vi "NI XNET CAN Signal Logger - Configure Dialog.vi"(8 "error in (no error)":errorcluster, 10 "CAN Configurations in":T1[](array[typedef]) {"Sample Rate (Hz)" format="%#_13g"}, 11 "LogSpec in":T2={"Log file folder"=path "C:/Users/NI/Desktop/Data", "Log file name"="LogFile_{Year}-{Month}-{Day}-{Hour}-{Minute}-{Second}.tdms", "Segment Files"=FALSE, "Segment File Size"=100} {"Segment File Size" format="%.0f MB"}) -> (0 "error out":errorcluster, 2 "CAN Configurations out":T1[](array[typedef]) {"Sample Rate (Hz)" format="%#_13g"}, 3 "LogSpec out":T2={"Log file folder"=path "C:/Users/NI/Desktop/Data", "Log file name"="LogFile_{Year}-{Month}-{Day}-{Hour}-{Minute}-{Second}.tdms", "Segment Files"=FALSE, "Segment File Size"=100} {"Segment File Size" format="%.0f MB"})   [LabVIEW 2021, in "XNET-CAN-Signal-Logger.lvlib"]
uses:
  XNET-CAN-Signal-Logger.lvlib
  Typedef/Def-CAN Port Configuration.ctl
  Typedef/Def-LogSpec.ctl
  <resource>/objmgr/xnet.rc
panel:
  in  "OK":bool
  in  "CAN Configurations":T1[](array[typedef]) {"Sample Rate (Hz)" format="%#_13g"}
  out "Preview":string caption="Preview:"
  in  "Log file name":string="LogFile_{Year}-{Month}-{Day}-{Hour}-{Minute}-{Second}.tdms"
  in  "Log file folder":path=path "C:/Users/NI/Desktop/Data"
  in  "Cancel":bool
  in  "Segment Files":bool=TRUE
  in  "Segment File Size":i64=100 caption="Seg File Size" format="%.0f MB"
  # "Configuration"
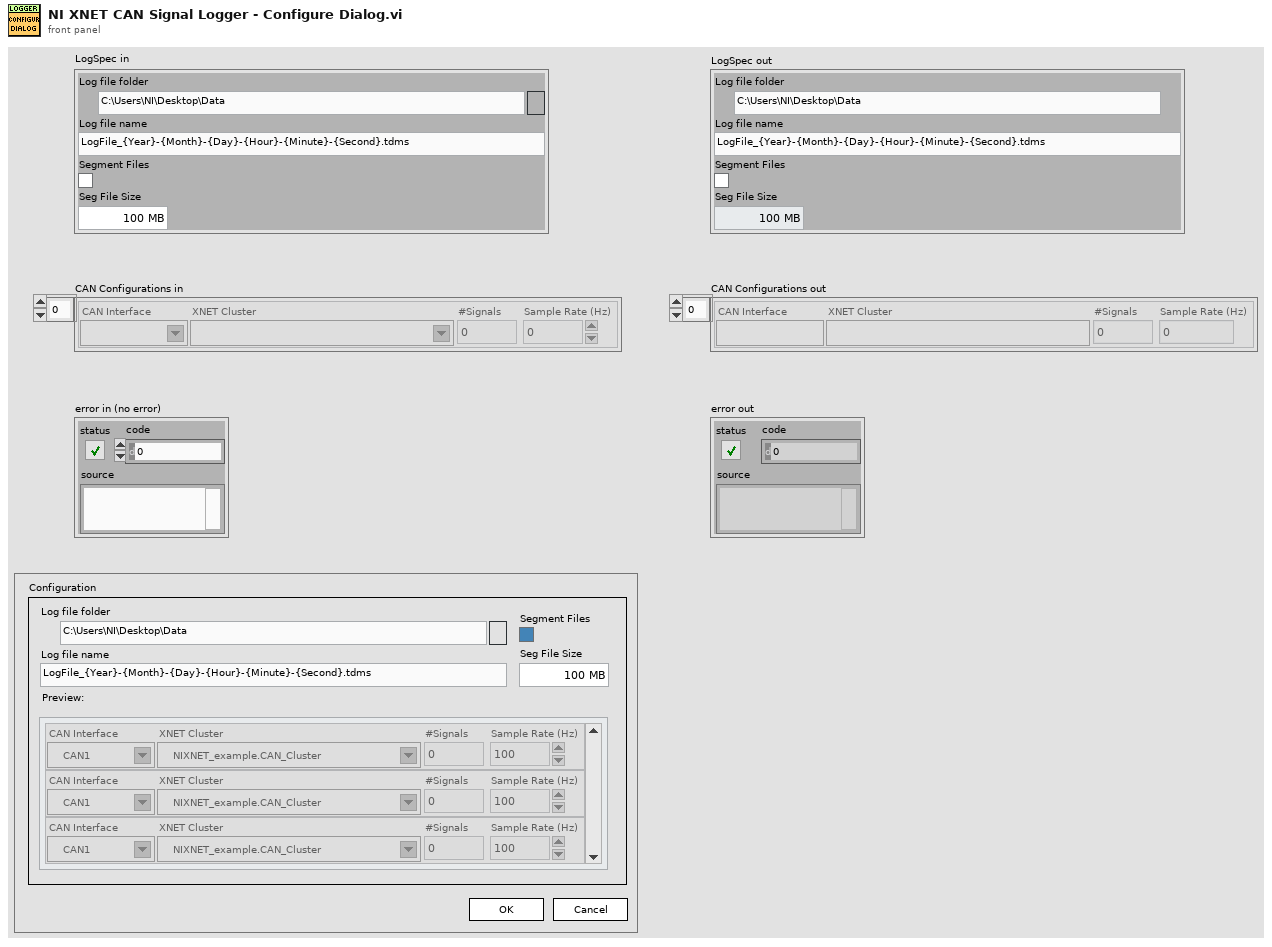
[diagram p1: front panel]
types:
  T1 = typedef "XNET-CAN-Signal-Logger.lvlib/Def-CAN Port Configuration.ctl" = cluster{"CAN Interface":refnum<k21>, "XNET Cluster":refnum<k21>, "#Signals":i32, "Sample Rate (Hz)":dbl}
  T2 = typedef "XNET-CAN-Signal-Logger.lvlib/Def-LogSpec.ctl" = cluster{"Log file folder":path, "Log file name":string, "Segment Files":bool, "Segment File Size":i64}
  T3 = enum32{"Invalid", "Standard", "Closed", "Hidden", "Minimized", "Maximized"}
  T4 = enum32{"invalid app kind", "Development System", "Run Time System", "Student Edition", "Embedded LabVIEW", "Evaluation", "Custom"}
  T5 = cluster{"Core":cluster{"Current VI Reference":refnum<vi>, "Close Panel on Exit?":bool}, "LogSpec in":T2, "CAN Configurations in":T1[]}
  T6 = cluster{"Current VI Reference":refnum<vi>, "Close Panel on Exit?":bool}
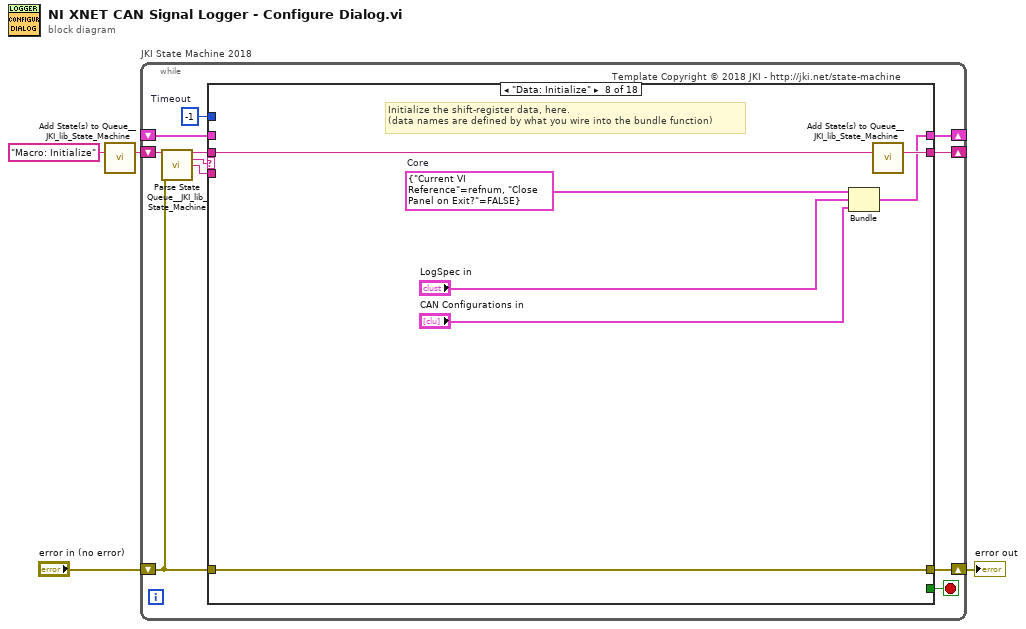
[diagram p0: block diagram]
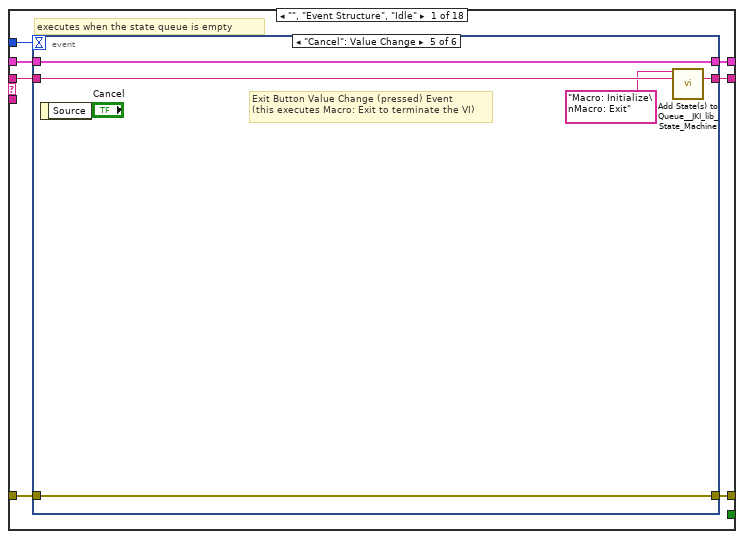
[diagram p2: hidden frame]
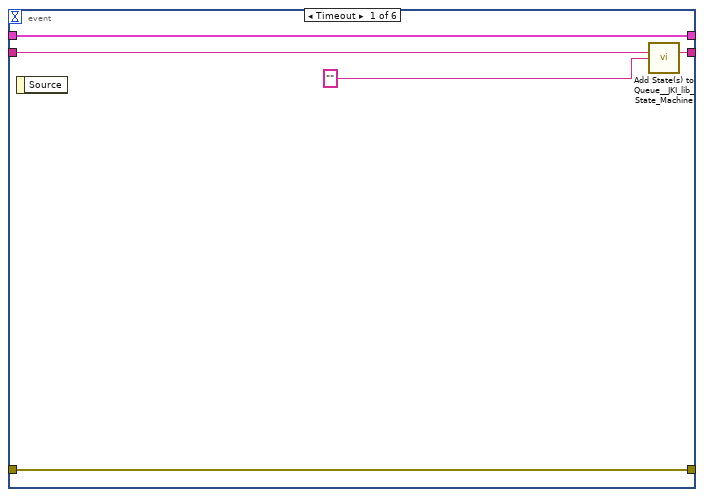
[diagram p3: hidden frame]
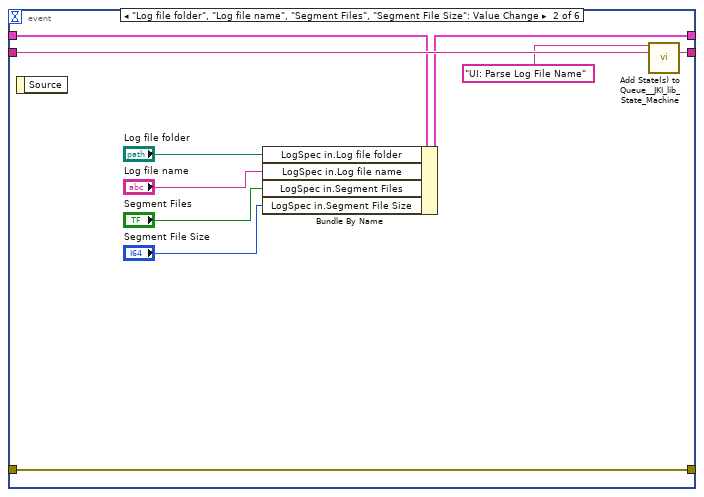
[diagram p4: hidden frame]
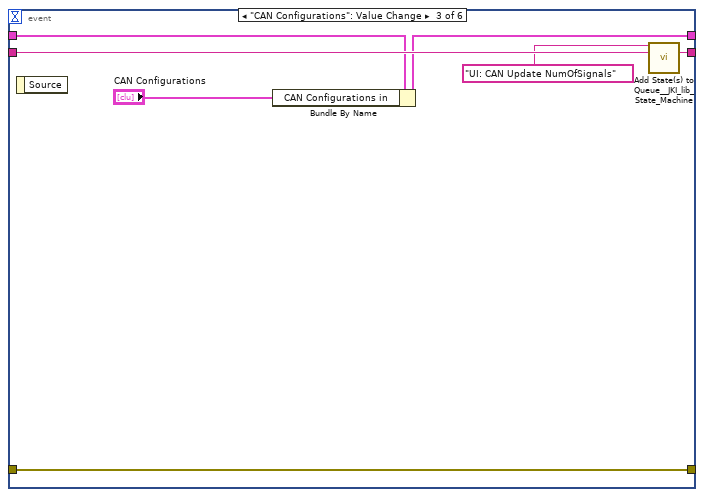
[diagram p5: hidden frame]
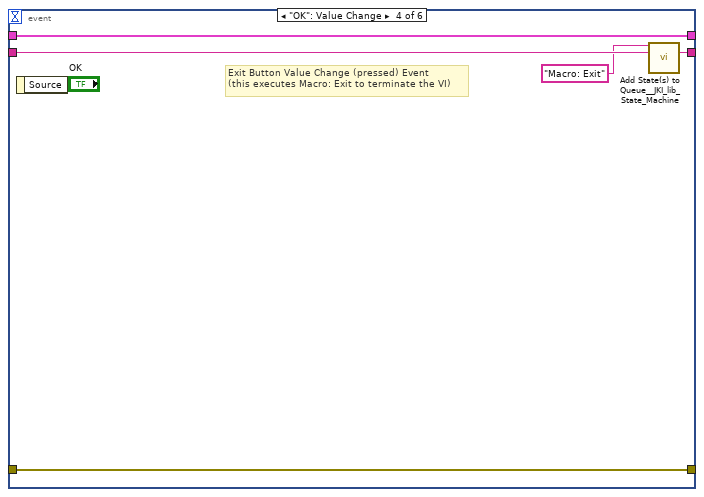
[diagram p6: hidden frame]
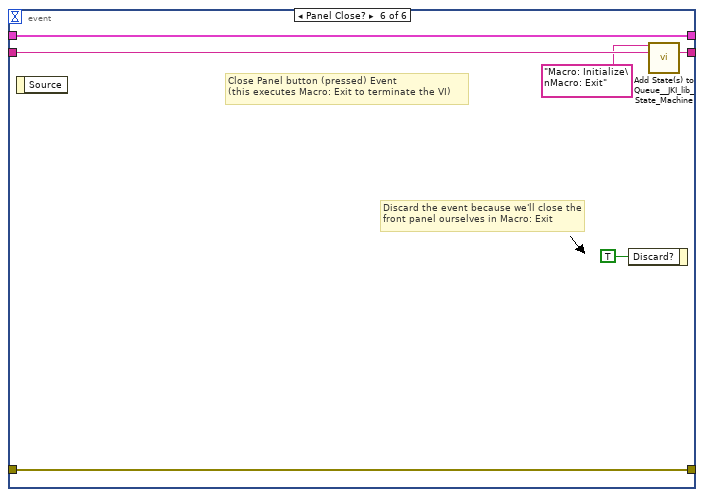
[diagram p7: hidden frame]
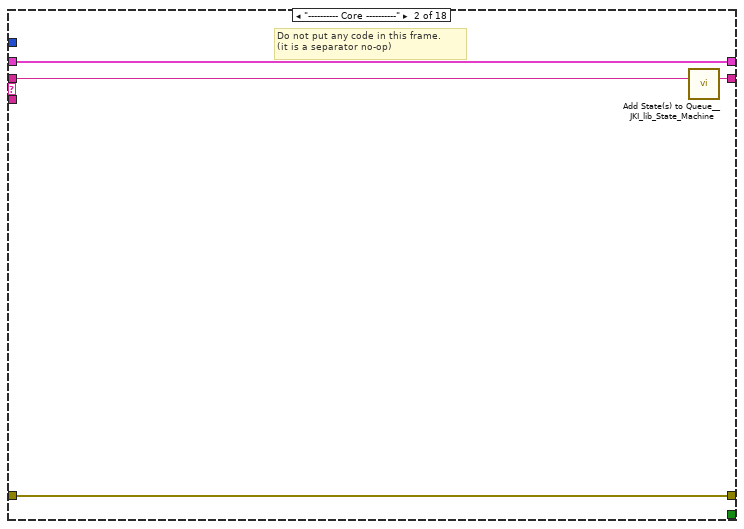
[diagram p8: hidden frame]
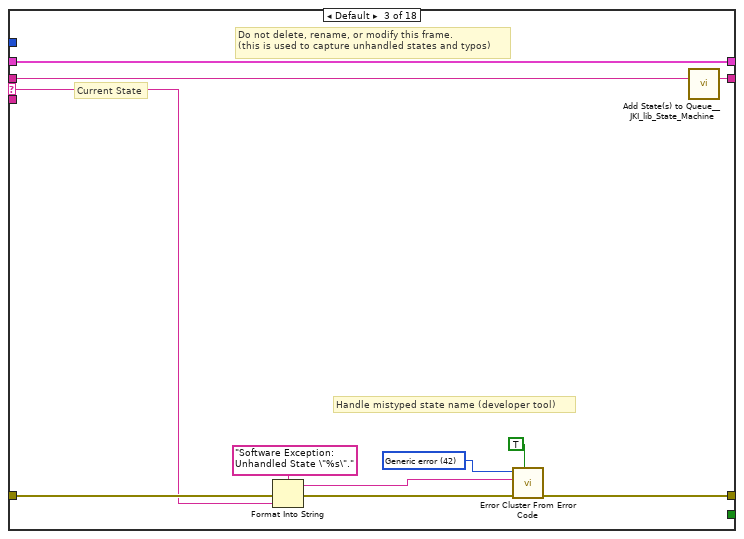
[diagram p9: hidden frame]
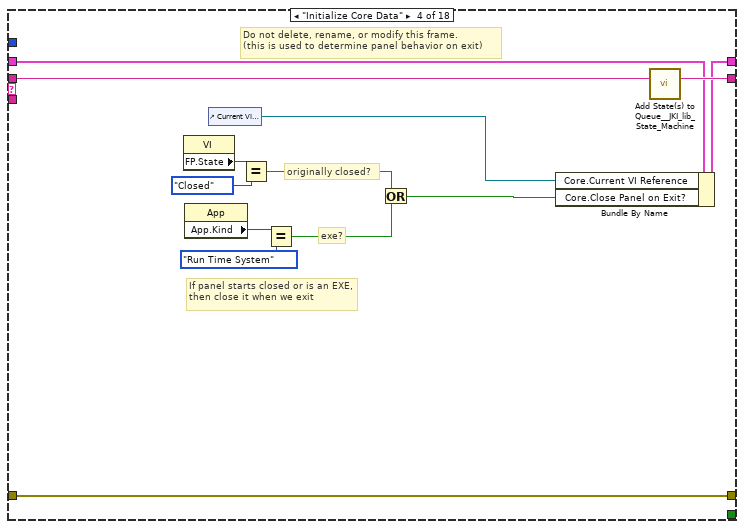
[diagram p10: hidden frame]
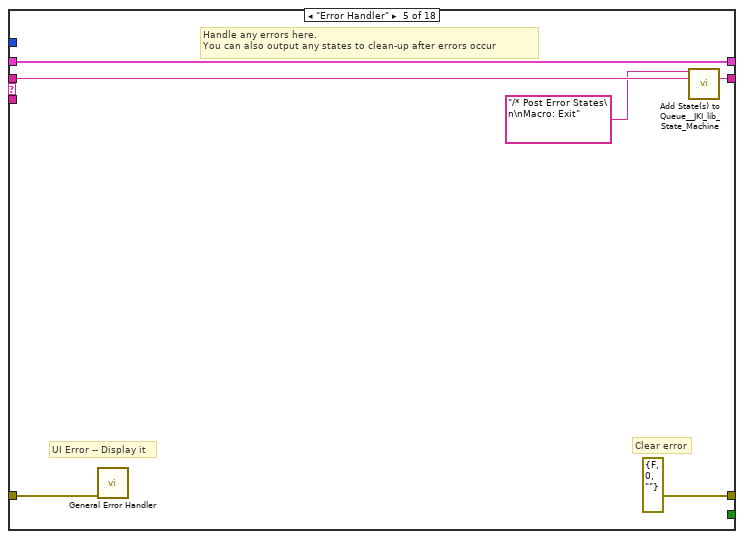
[diagram p11: hidden frame]
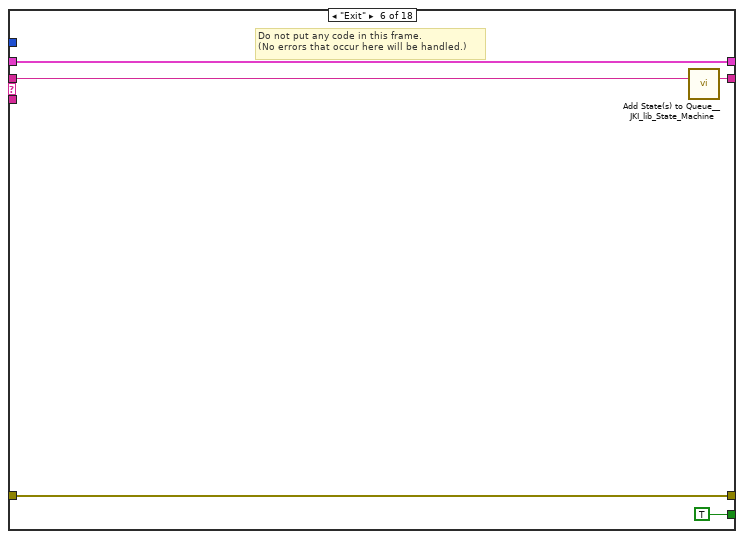
[diagram p12: hidden frame]
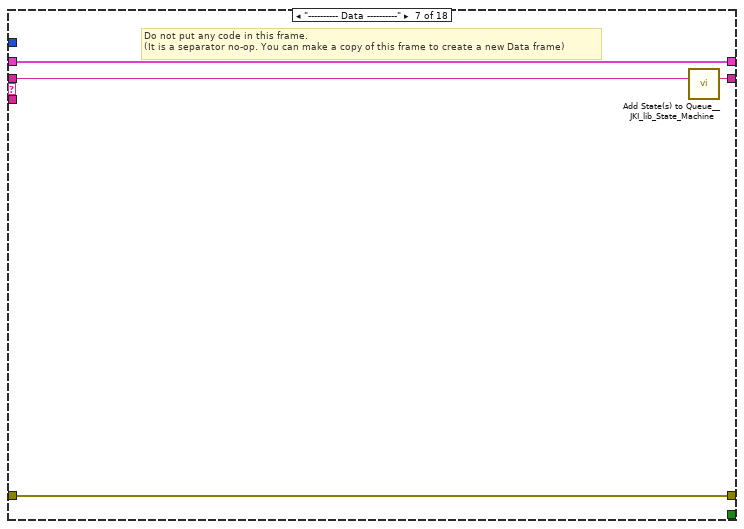
[diagram p13: hidden frame]
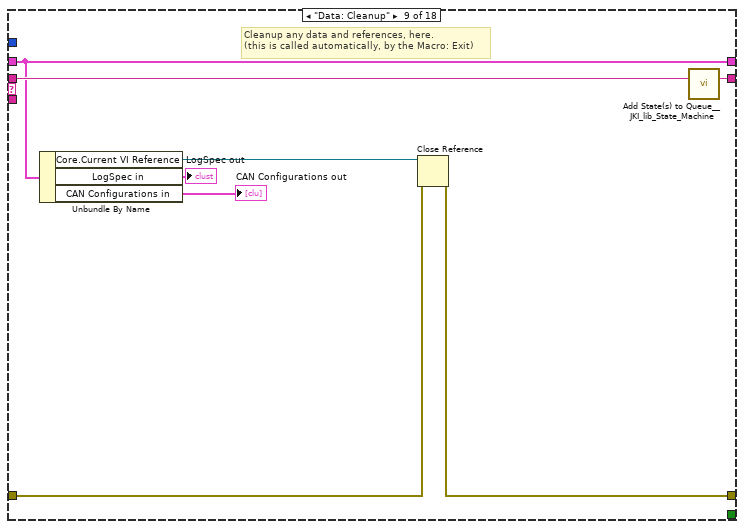
[diagram p14: hidden frame]
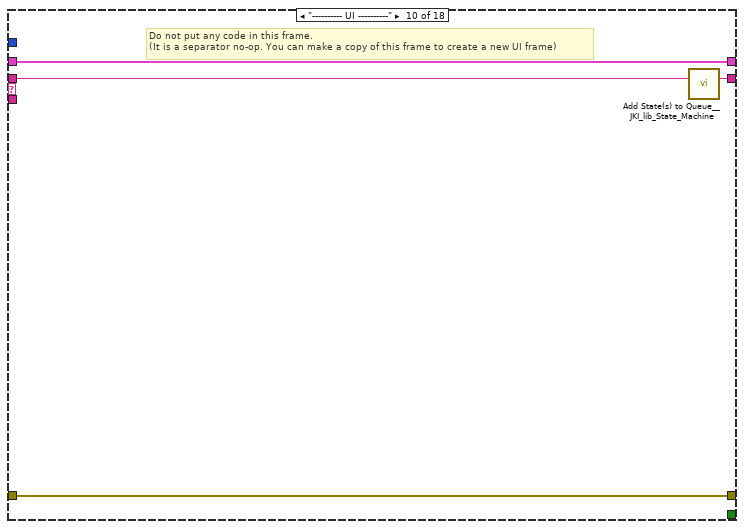
[diagram p15: hidden frame]
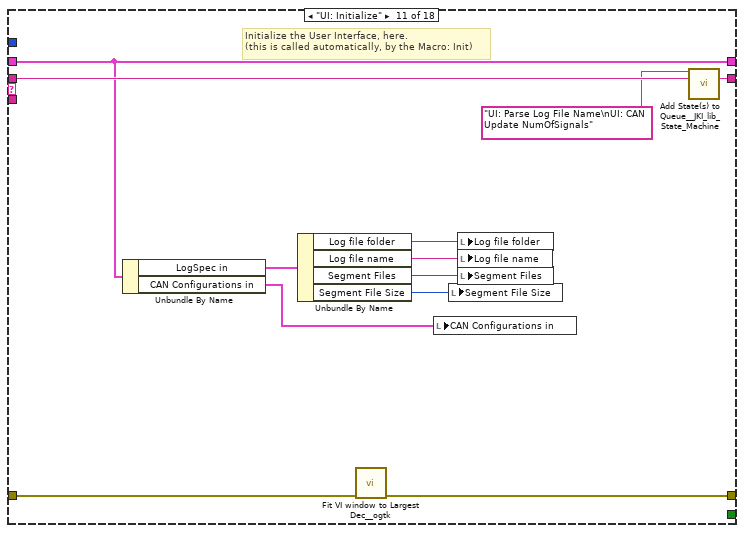
[diagram p16: hidden frame]
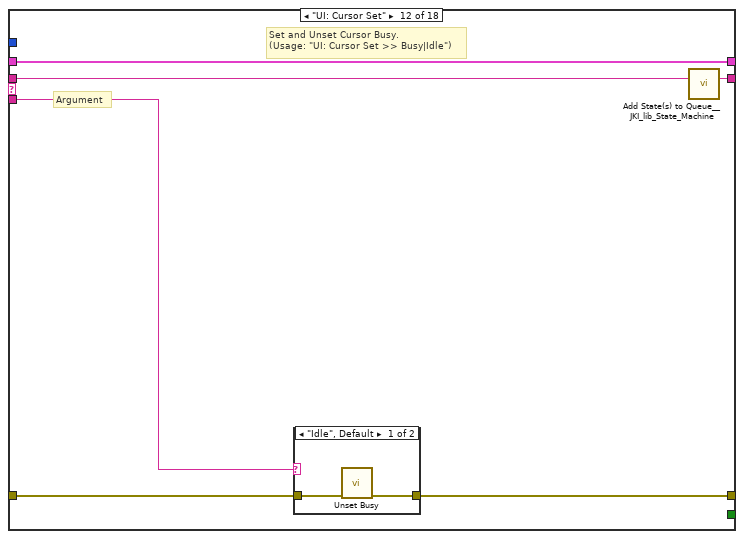
[diagram p17: hidden frame]
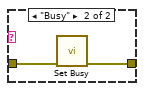
[diagram p18: hidden frame]
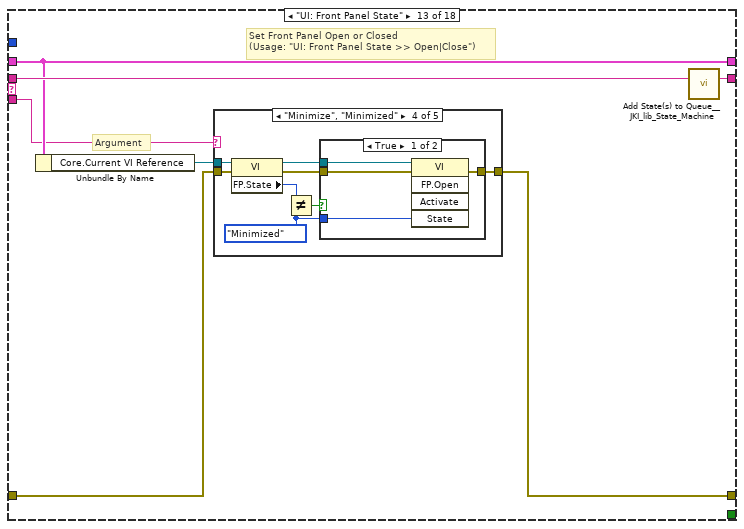
[diagram p19: hidden frame]
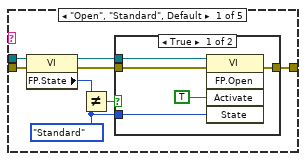
[diagram p20: hidden frame]
diagram:
  n1 = call <vilib>:"Add State(s) to Queue__JKI_lib_State_Machine.vi"("State(s) in (\"\")"="Macro: Initialize") -> ("States Out"=w4:string)  [unwired: 14 in]
  n2 = while "JKI State Machine 2018" {
    shift-right: [w8] -> _
    shift-left: _ -> [w7]
    shift-right: [w11] -> w1
    shift-left: "error in (no error)" -> [w5]
    shift-right: [w10] -> _
    shift-left: w4 -> [w12]
    stop <- w9 stop-if-true
    w6 = -1  # Timeout
    # "Template Copyright © 2018 JKI - http://jki.net/state-machine"
    n3 = call <vilib>:"Parse State Queue__JKI_lib_State_Machine.vi"("State Queue"=w12, "Error In (no error)"=w5) -> ("Remaining States"=w14:string, "Current State"=w15:string, "Arguments"=w13:string)  [unwired: 11 in]
    n4 = case shown="\"Data: Initialize\"" w15 {
      selector: w15 -> [_ _ w65 _ _ _ _ _ _ _ _ _ _ _ _ _ _ _]
      tunnel: w14 -> [w22 w64 w69 w88 w94 w99 w103 w110 w118 w122 w134 w140 w151 w222 w229 w238 w243 w253]
      tunnel: w13 -> [_ _ _ _ _ _ _ _ _ _ _ w135 w145 _ _ _ _ _]
      tunnel: w7 -> [w20 w61 w67 w81 w91 w97 w100 _ w113 w119 w126 w138 w147 w218 w224 w235 w240 w250]
      tunnel: [w19 w62 w71 w85 errorcluster {"status"=FALSE, "code"=0, "source"=""} ("error out") w96 w101 w107 w114 w120 w123 w136 w148 w220 w227 w236 w241 w251] -> w11
      tunnel: w5 -> [w18 w62 w70 w85 w90 w96 w101 w107 w115 w120 w132 w137 w149 w220 w227 w236 w241 w251]
      tunnel: [w21 w63 w68 w87 w93 w98 w102 w109 w117 w121 w133 w139 w150 w221 w228 w237 w242 w252] -> w10
      tunnel: [_ _ _ _ _ TRUE _ _ _ _ _ _ _ _ _ _ _ _] -> w9
      tunnel: [w17 w61 w67 w86 w91 w97 w100 w108 w113 w119 w126 w138 w147 w218 w226 w235 w240 w250] -> w8
      tunnel: w6 -> [w16 _ _ _ _ _ _ _ _ _ _ _ _ _ _ _ _ _]
      frame "", "Event Structure", "Idle" {
        # "executes when the state queue is empty"
        n5 = event shown="[4] \"Cancel\": Value Change" {
          selector: _ -> [_ _ _ _ _ _]
          dyn-events: _ -> [_ _ _ _ _ _]
          timeout: w16 -> [_ _ _ _ _ _]
          tunnel: w22 -> [w24 w37 w44 w49 w54 w60]
          tunnel: [w27 w36 w43 w48 w53 w59] -> w21
          tunnel: w20 -> [w25 w34 w41 w46 w51 w57]
          tunnel: [w26 w35 w42 w47 w52 w58] -> w19
          tunnel: w18 -> [w26 w35 w42 w47 w52 w58]
          tunnel: [w25 w32 w39 w46 w51 w57] -> w17
          event Timeout {
            n6 = event-data() -> ()  [unwired: 1 in, 1 out]
            n7 = call <vilib>:"Add State(s) to Queue__JKI_lib_State_Machine.vi"("State(s) in (\"\")"=w24, "State(s) at Back (\"\")"="" ("string")) -> ("States Out"=w27:string)  [unwired: 13 in]
          }
          event "Log file folder", "Log file name", "Segment Files", "Segment File Size": Value Change {
            n8 = event-data() -> ()  [unwired: 1 in, 1 out]
            n9 = Bundle By Name(cluster=w34, "LogSpec in.Log file folder"="Log file folder", "LogSpec in.Log file name"="Log file name", "LogSpec in.Segment Files"="Segment Files", "LogSpec in.Segment File Size"="Segment File Size") -> (w32:T5)
            n10 = call <vilib>:"Add State(s) to Queue__JKI_lib_State_Machine.vi"("State(s) in Front (\"\")"="UI: Parse Log File Name", "State(s) in (\"\")"=w37) -> ("States Out"=w36:string)  [unwired: 13 in]
          }
          event "CAN Configurations": Value Change {
            n11 = event-data() -> ()  [unwired: 1 in, 1 out]
            n12 = Bundle By Name(cluster=w41, "CAN Configurations in"="CAN Configurations") -> (w39:T5)
            n13 = call <vilib>:"Add State(s) to Queue__JKI_lib_State_Machine.vi"("State(s) in Front (\"\")"="UI: CAN Update NumOfSignals", "State(s) in (\"\")"=w44) -> ("States Out"=w43:string)  [unwired: 13 in]
          }
          event "OK": Value Change {
            # "Exit Button Value Change (pressed) Event\n(this executes Macro: Exit to terminate the VI)"
            n14 = event-data() -> ()  [unwired: 1 in, 1 out]
            n15 = call <vilib>:"Add State(s) to Queue__JKI_lib_State_Machine.vi"("State(s) in Front (\"\")"="Macro: Exit", "State(s) in (\"\")"=w49) -> ("States Out"=w48:string)  [unwired: 13 in]
          }
          event "Cancel": Value Change {
            # "Exit Button Value Change (pressed) Event\n(this executes Macro: Exit to terminate the VI)"
            n16 = event-data() -> ()  [unwired: 1 in, 1 out]
            n17 = call <vilib>:"Add State(s) to Queue__JKI_lib_State_Machine.vi"("State(s) in Front (\"\")"="Macro: Initialize\nMacro: Exit", "State(s) in (\"\")"=w54) -> ("States Out"=w53:string)  [unwired: 13 in]
          }
          event Panel Close? {
            # "Discard the event because we'll close the front panel ourselves in Macro: Exit"
            # "Close Panel button (pressed) Event\n(this executes Macro: Exit to terminate the VI)"
            n18 = event-data() -> ()  [unwired: 1 in, 1 out]
            n19 = event-data("Discard?"=TRUE) -> ()  [unwired: 1 in, 1 out]
            n20 = call <vilib>:"Add State(s) to Queue__JKI_lib_State_Machine.vi"("State(s) in Front (\"\")"="Macro: Initialize\nMacro: Exit", "State(s) in (\"\")"=w60) -> ("States Out"=w59:string)  [unwired: 13 in]
          }
        }
      }
      frame "---------- Core ----------" {
        # "Do not put any code in this frame.\n(it is a separator no-op)"
        n21 = call <vilib>:"Add State(s) to Queue__JKI_lib_State_Machine.vi"("State(s) in (\"\")"=w64) -> ("States Out"=w63:string)  [unwired: 14 in]
      }
      frame Default {
        w74 = 42 items=["No error", "Argument error", "Memory is full", "Out of zone", "End of file", "File already open", "Generic file I/O error", "File not found", "File permission error", "Disk is full", "Duplicate path", "Too many files open", "System feature not enabled", "Resource file not found", "Cannot add resource", "Resource not found", "Image not found", "Image memory error", "Pen does not exist", "Config type invalid", "Config token not found", "Config parse error", "Config memory error", "Bad external code format", "Bad external code offset", "External code not present", "Null window", "Destroy window error", "Null menu", "Print aborted", "Bad print record", "Print driver error", "Windows error during printing", "Memory error during printing", "Print dialog error", "Generic print error", "Invalid device refnum", "Device not found", "Device parameter error", "Device unit error", "Cannot open device", "Device call aborted", "Generic error", "Cancelled by user", "Object ID too low", "Object ID too high", "Object not in heap", "Unknown heap", "Unknown object (invalid DefProc)", "Unknown object (DefProc not in table)", "Message out of range", "Invalid (null) method", "Unknown message", "Manager call not supported", "Bad address", "Network operation in progress", "Network operation timed out", "Connection is busy", "Network attribute not supported", "Network error", "Address in use", "System out of memory", "Connection aborted", "Connection refused", "Not connected", "Already connected", "Connection closed", "Initialization error (interapplication manager)", "Bad occurrence", "Wait on unbound occurrence handler", "Occurrence queue overflow", "Datalog type conflict", "Unused", "Unrecognized type (interapplication manager)", "Memory corrupt", "Failed to make temporary DLL", "Old CIN version", "Drag socket not found", "Failed to load drop-object", "Failed to register OLE object", "Failed to release OLE object", "Format specifier type mismatch", "Unknown format specifier", "Too few format specifiers", "Too many format specifiers", "Scan failed", "Newer CIN version", "Error converting to variant", "Runtime menu error", "Password tampered", "Variant attribute not found", "Incompatible variant data type", "Event data is not available", "Event Store is not present", "Occurrence is not found", "Event Queue is not created", "Event info is not available", "Refnum passed is NULL", "Error retrieving Class GUID", "Error retrieving CoClass GUID", "Error retrieving TypeLib GUID.", "Bad built application magic bytes.", "Specific driver is different from the specific driver associated with the Logical Name.", "There is no session opened to the class driver.", "Max Error", "MAX - Error with config objects", "MAX - Error loading configuration", "MAX - Group not supported"]
        # "Current State"
        # "Do not delete, rename, or modify this frame.\n(this is used to capture unhandled states and typos)"
        # "Handle mistyped state name (developer tool)"
        n22 = Format Into String(format string="Software Exception: Unhandled State \"%s\"." ("message"), error in=w70, w65) -> (resulting string=w73:string, error out=w72:errorcluster)  [unwired: 1 in]
        n23 = call <vilib>:"Error Cluster From Error Code.vi"("show call chain? (False)"=TRUE, "error in (no error)"=w72, "error message (\"\")"=w73, "error code (0)"=w74) -> ("error out"=w71:errorcluster)  [unwired: 5 in]
        n24 = call <vilib>:"Add State(s) to Queue__JKI_lib_State_Machine.vi"("State(s) in (\"\")"=w69) -> ("States Out"=w68:string)  [unwired: 14 in]
      }
      frame "Initialize Core Data" {
        # "Do not delete, rename, or modify this frame.\n(this is used to determine panel behavior on exit)"
        # "originally closed?"
        # "exe?"
        # "If panel starts closed or is an EXE, then close it when we exit"
        n25 = property class="VI"() -> ("FP.State"=w78:T3)  [unwired: 2 in, 2 out]
        n26 = property class="App"() -> ("App.Kind"=w84:T4)  [unwired: 2 in, 2 out]
        n27 = control-ref of="Current VI Reference"() -> (w79:refnum<vi>)
        n28 = Equal?(x=w78, y=T3."Closed" ("Front Panel Window:State")) -> (x = y?=w76:bool)
        n29 = Equal?(x=w84, y=T4."Run Time System" ("Application:Kind")) -> (x = y?=w82:bool)
        n30 = Or(x=w76, y=w82) -> (x .or. y?=w80:bool)
        n31 = Bundle By Name(cluster=w81, "Core.Current VI Reference"=w79, "Core.Close Panel on Exit?"=w80) -> (w86:T5)
        n32 = call <vilib>:"Add State(s) to Queue__JKI_lib_State_Machine.vi"("State(s) in (\"\")"=w88) -> ("States Out"=w87:string)  [unwired: 14 in]
      }
      frame "Error Handler" {
        # "UI Error -- Display it"
        # "Handle any errors here.\nYou can also output any states to clean-up after errors occur"
        # "Clear error"
        n33 = call <vilib>:"General Error Handler.vi"("error in (no error)"=w90) -> ()  [unwired: 10 in, 5 out]
        n34 = call <vilib>:"Add State(s) to Queue__JKI_lib_State_Machine.vi"("State(s) in Front (\"\")"="/* Post Error States\n\nMacro: Exit", "State(s) in (\"\")"=w94) -> ("States Out"=w93:string)  [unwired: 13 in]
      }
      frame "Exit" {
        # "Do not put any code in this frame.\n(No errors that occur here will be handled.)"
        n35 = call <vilib>:"Add State(s) to Queue__JKI_lib_State_Machine.vi"("State(s) in (\"\")"=w99) -> ("States Out"=w98:string)  [unwired: 14 in]
      }
      frame "---------- Data ----------" {
        # "Do not put any code in this frame.\n(It is a separator no-op. You can make a copy of this frame to create a new Data frame)"
        n36 = call <vilib>:"Add State(s) to Queue__JKI_lib_State_Machine.vi"("State(s) in (\"\")"=w103) -> ("States Out"=w102:string)  [unwired: 14 in]
      }
      frame "Data: Initialize" {
        w106 = T6 {"Current VI Reference"=refnum, "Close Panel on Exit?"=FALSE}  # Core
        # "Initialize the shift-register data, here.\n(data names are defined by what you wire into the bundle function)"
        n37 = Bundle("Core"=w106, "LogSpec in"="LogSpec in", "CAN Configurations in"="CAN Configurations in") -> (w108:T5)  [unwired: 1 in]
        n38 = call <vilib>:"Add State(s) to Queue__JKI_lib_State_Machine.vi"("State(s) in (\"\")"=w110) -> ("States Out"=w109:string)  [unwired: 14 in]
      }
      frame "Data: Cleanup" {
        # "Cleanup any data and references, here.\n(this is called automatically, by the Macro: Exit)"
        n39 = Unbundle By Name(w113) -> ("Core.Current VI Reference"=w116:refnum<vi>, "LogSpec in"=→"LogSpec out":T2, "CAN Configurations in"=→"CAN Configurations out":T1[])
        n40 = Close Reference(reference=w116, error in (no error)=w115) -> (error out=w114:errorcluster)
        n41 = call <vilib>:"Add State(s) to Queue__JKI_lib_State_Machine.vi"("State(s) in (\"\")"=w118) -> ("States Out"=w117:string)  [unwired: 14 in]
      }
      frame "---------- UI ----------" {
        # "Do not put any code in this frame.\n(It is a separator no-op. You can make a copy of this frame to create a new UI frame)"
        n42 = call <vilib>:"Add State(s) to Queue__JKI_lib_State_Machine.vi"("State(s) in (\"\")"=w122) -> ("States Out"=w121:string)  [unwired: 14 in]
      }
      frame "UI: Initialize" {
        # "Initialize the User Interface, here.\n(this is called automatically, by the Macro: Init)"
        n43 = Unbundle By Name(w126) -> ("LogSpec in"=w125:T2, "CAN Configurations in"=w124:T1[])
        n44 = Unbundle By Name(w125) -> ("Log file folder"=w130:path, "Log file name"=w129:string, "Segment Files"=w128:bool, "Segment File Size"=w127:i64)
        n45 = call <userlib>:"Fit VI window to Largest Dec__ogtk.vi"("error in (no error)"=w132) -> ("error out"=w123:errorcluster)  [unwired: 5 in, 1 out]
        n46 = local write "CAN Configurations in"(w124) -> ()
        n47 = local write "Segment File Size"(w127) -> ()
        n48 = local write "Log file folder"(w130) -> ()
        n49 = local write "Log file name"(w129) -> ()
        n50 = local write "Segment Files"(w128) -> ()
        n51 = call <vilib>:"Add State(s) to Queue__JKI_lib_State_Machine.vi"("State(s) in Front (\"\")"="UI: Parse Log File Name\nUI: CAN Update NumOfSignals" ("State(s) in Front (\"\")"), "State(s) in (\"\")"=w134) -> ("States Out"=w133:string)  [unwired: 13 in]
      }
      frame "UI: Cursor Set" {
        # "Argument"
        # "Set and Unset Cursor Busy.\n(Usage: \"UI: Cursor Set >> Busy|Idle\")"
        n52 = case shown="\"Idle\", Default" w135 {
          tunnel: w137 -> [w142 w144]
          tunnel: [w141 w143] -> w136
          frame "Idle", Default {
            n53 = call <vilib>:"Unset Busy.vi"("error in (no error)"=w142) -> ("error out"=w141:errorcluster)  [unwired: 10 in]
          }
          frame "Busy" {
            n54 = call <vilib>:"Set Busy.vi"("error in (no error)"=w144) -> ("error out"=w143:errorcluster)  [unwired: 9 in, 1 out]
          }
        }
        n55 = call <vilib>:"Add State(s) to Queue__JKI_lib_State_Machine.vi"("State(s) in (\"\")"=w140) -> ("States Out"=w139:string)  [unwired: 14 in]
      }
      frame "UI: Front Panel State" {
        # "Argument"
        # "Set Front Panel Open or Closed\n(Usage: \"UI: Front Panel State >> Open|Close\")"
        n56 = Unbundle By Name(w147) -> ("Core.Current VI Reference"=w146:refnum<vi>)
        n57 = case shown="\"Minimize\", \"Minimized\"" w145 {
          tunnel: w149 -> [w157 w172 w183 w196 w209]
          tunnel: [w159 w173 w185 w198 w211] -> w148
          tunnel: w146 -> [w158 w170 w184 w197 w210]
          frame "Open", "Standard", Default {
            w152 = T3."Standard" ("State")
            n58 = property class="VI"(reference=w158, error in=w157) -> (reference out=w155:refnum<vi>, error out=w156:errorcluster, "FP.State"=w154:T3)
            n59 = Not Equal?(x=w154, y=w152) -> (x != y?=w153:bool)
            n60 = case shown="True" w153 {
              tunnel: [w163 w165] -> w159
              tunnel: w156 -> [w162 w165]
              tunnel: w155 -> [w161 _]
              tunnel: w152 -> [w160 _]
              frame True {
                n61 = invoke class="VI" method="FP.Open"(reference=w161, error in=w162, "Activate"=TRUE, "State"=w160) -> (error out=w163:errorcluster)  [unwired: 1 in, 4 out]
              }
              frame False {
              }
            }
          }
          frame "Close", "Closed" {
            n62 = property class="VI"(reference=w170, error in=w172) -> (reference out=w169:refnum<vi>, error out=w171:errorcluster, "FP.State"=w167:T3)
            n63 = Not Equal?(x=w167, y=T3."Closed" ("Front Panel Window:State")) -> (x != y?=w166:bool)
            n64 = case shown="True" w166 {
              tunnel: [w174 w177] -> w173
              tunnel: w171 -> [w174 w176]
              tunnel: w169 -> [_ w175]
              frame False {
              }
              frame True {
                n65 = invoke class="VI" method="FP.Close"(reference=w175, error in=w176) -> (error out=w177:errorcluster)  [unwired: 1 in, 2 out]
              }
            }
          }
          frame "Hidden", "Hide" {
            w178 = T3."Hidden" ("State")
            n66 = property class="VI"(reference=w184, error in=w183) -> (reference out=w181:refnum<vi>, error out=w182:errorcluster, "FP.State"=w180:T3)
            n67 = Not Equal?(x=w180, y=w178) -> (x != y?=w179:bool)
            n68 = case shown="True" w179 {
              tunnel: [w189 w190] -> w185
              tunnel: w182 -> [w188 w190]
              tunnel: w181 -> [w187 _]
              tunnel: w178 -> [w186 _]
              frame True {
                n69 = invoke class="VI" method="FP.Open"(reference=w187, error in=w188, "State"=w186) -> (error out=w189:errorcluster)  [unwired: 2 in, 4 out]
              }
              frame False {
              }
            }
          }
          frame "Minimize", "Minimized" {
            w191 = T3."Minimized" ("State")
            n70 = property class="VI"(reference=w197, error in=w196) -> (reference out=w194:refnum<vi>, error out=w195:errorcluster, "FP.State"=w193:T3)
            n71 = Not Equal?(x=w193, y=w191) -> (x != y?=w192:bool)
            n72 = case shown="True" w192 {
              tunnel: [w202 w203] -> w198
              tunnel: w195 -> [w201 w203]
              tunnel: w194 -> [w200 _]
              tunnel: w191 -> [w199 _]
              frame True {
                n73 = invoke class="VI" method="FP.Open"(reference=w200, error in=w201, "State"=w199) -> (error out=w202:errorcluster)  [unwired: 2 in, 4 out]
              }
              frame False {
              }
            }
          }
          frame "Maximize", "Maximized" {
            w204 = T3."Maximized" ("State")
            n74 = property class="VI"(reference=w210, error in=w209) -> (reference out=w207:refnum<vi>, error out=w208:errorcluster, "FP.State"=w206:T3)
            n75 = Not Equal?(x=w206, y=w204) -> (x != y?=w205:bool)
            n76 = case shown="True" w205 {
              tunnel: [w215 w216] -> w211
              tunnel: w208 -> [w214 w216]
              tunnel: w207 -> [w213 _]
              tunnel: w204 -> [w212 _]
              frame True {
                n77 = invoke class="VI" method="FP.Open"(reference=w213, error in=w214, "State"=w212) -> (error out=w215:errorcluster)  [unwired: 2 in, 4 out]
              }
              frame False {
              }
            }
          }
        }
        n78 = call <vilib>:"Add State(s) to Queue__JKI_lib_State_Machine.vi"("State(s) in (\"\")"=w151) -> ("States Out"=w150:string)  [unwired: 14 in]
      }
      frame "UI: Parse Log File Name" {
        n79 = Unbundle By Name(w218) -> ("LogSpec in.Log file name"=w217:string)
        n80 = call "Parse Log File Name.vi"("Log file name"=w217) -> ("Parsed Log file name"=→"Preview":string)  [unwired: 10 in]
        n81 = call <vilib>:"Add State(s) to Queue__JKI_lib_State_Machine.vi"("State(s) in (\"\")"=w222) -> ("States Out"=w221:string)  [unwired: 14 in]
      }
      frame "UI: CAN Update NumOfSignals" {
        n82 = Unbundle By Name(w224) -> ("CAN Configurations in"=w223:T1[])
        n83 = for {
          tunnel: w223 -> [w232] mode=indexing
          tunnel: [w230] -> w225 mode=indexing
          n84 = Unbundle By Name(w232) -> ("XNET Cluster"=w234:refnum<k21>)
          n85 = property class="XNET Cluster"(reference=w234) -> ("Sigs"=w233:refnum<k21>[])  [unwired: 1 in, 2 out]
          n86 = Array Size(array=w233) -> (size(s)=w231:i32)
          n87 = Bundle By Name(cluster=w232, "#Signals"=w231) -> (w230:T1)
        }
        n88 = Bundle By Name(cluster=w224, "CAN Configurations in"=w225) -> (w226:T5)
        n89 = local write "CAN Configurations"(w225) -> ()
        n90 = call <vilib>:"Add State(s) to Queue__JKI_lib_State_Machine.vi"("State(s) in (\"\")"=w229) -> ("States Out"=w228:string)  [unwired: 14 in]
      }
      frame "---------- Macro ----------" {
        # "Do not put any code in this frame.\n(It is a separator no-op. You can make a copy of this frame to create a new Macro frame)"
        n91 = call <vilib>:"Add State(s) to Queue__JKI_lib_State_Machine.vi"("State(s) in (\"\")"=w238) -> ("States Out"=w237:string)  [unwired: 14 in]
      }
      frame "Macro: Initialize" {
        # "Initialization Macro\n(This is called once, when the VI starts)"
        n92 = call <vilib>:"Add State(s) to Queue__JKI_lib_State_Machine.vi"("State(s) in Front (\"\")"="Data: Initialize\nInitialize Core Data\n\nUI: Initialize\nUI: Front Panel State >> Open", "State(s) in (\"\")"=w243) -> ("States Out"=w242:string)  [unwired: 13 in]
      }
      frame "Macro: Exit" {
        # "Exit Macro\n(This is called once, when the VI exits)"
        n93 = Unbundle By Name(w250) -> ("Core.Close Panel on Exit?"=w249:bool)
        n94 = Select(t="UI: Front Panel State >> Close", s=w249, f="") -> (s? t:f=w246:string)
        n95 = call <vilib>:"Add State(s) to Queue__JKI_lib_State_Machine.vi"("State(s) in (\"\")"=w246, "State(s) at Back (\"\")"="Data: Cleanup\n\nExit") -> ("States Out"=w244:string)  [unwired: 13 in]
        n96 = call <vilib>:"Add State(s) to Queue__JKI_lib_State_Machine.vi"("State(s) in Front (\"\")"=w244, "State(s) in (\"\")"=w253) -> ("States Out"=w252:string)  [unwired: 13 in]
      }
    }
  }
  "error out" <- w1
